vi "Indexer Closed Loop Control.vi"() -> ()   [LabVIEW 2011]
panel:
  in  "D":dbl
  in  "I":dbl
  in  "P":dbl
  out "RPM Error":dbl
  out "Encoder Set Speed":dbl
  out "Actual Encoder Speed":dbl
  in  "Indexer Enabled":bool
  out "Output PWM":dbl
  in  "Decrement":bool
  in  "Increment":bool
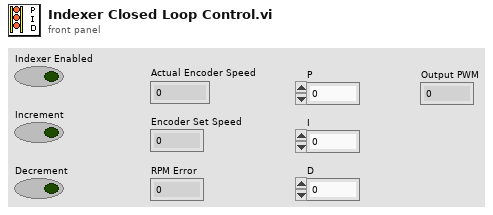
[diagram p1: front panel]
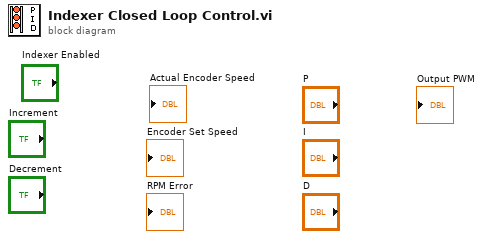
[diagram p0: block diagram]
diagram:
